vi "GetHWI.vi"(0 "NI Card in":refnum<class "NI Card.lvclass">, 11 "error in (no error)":errorcluster) -> (4 "NI Card out":refnum<class "NI Card.lvclass">, 6 "NI Card Hardware Image":T2, 8 "Parsed data":T1(array[cluster]), 15 "error out":errorcluster)   [LabVIEW 2013, in "NI Card.lvclass"]
uses:
  NI Card.lvclass
  NI Card.lvclass/NI Card.ctl
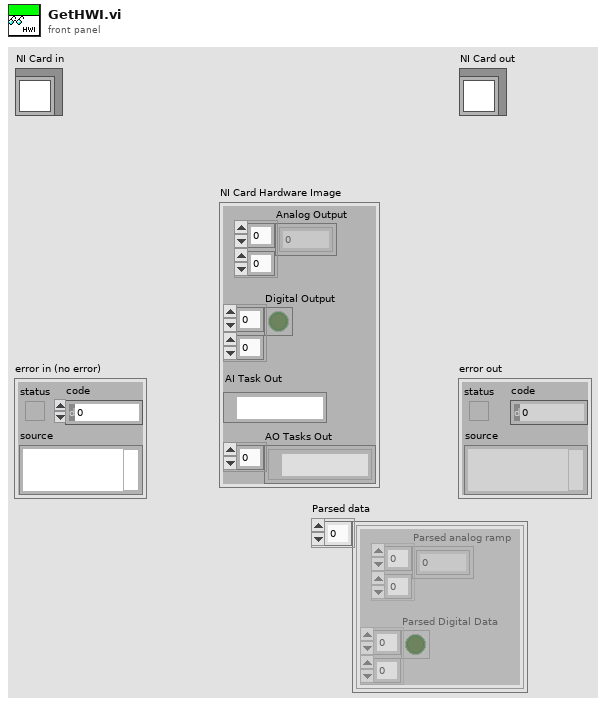
[diagram p1: front panel]
types:
  T1 = cluster{"Parsed analog ramp":dbl[][], "Parsed Digital Data":bool[][]}[]
  T2 = cluster{"Analog Output ":dbl[][], "Digital Output":bool[][], "AI Task Out":refnum<k21>, "AO Tasks Out":refnum<k21>[]}
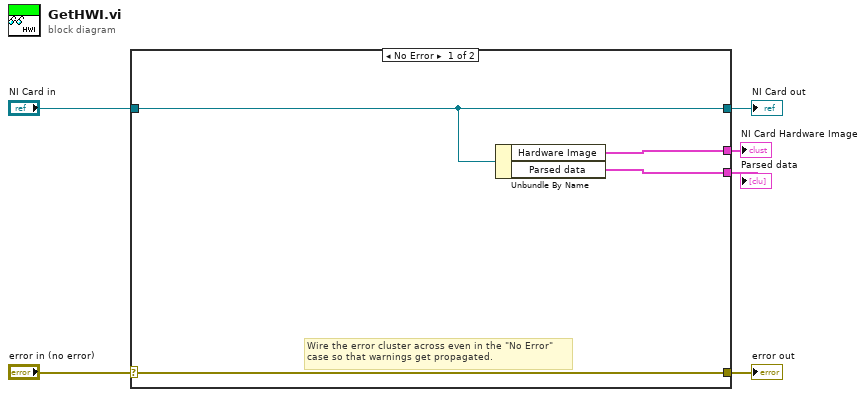
[diagram p0: block diagram]
diagram:
  n1 = case shown="No Error" "error in (no error)" {
    selector: "error in (no error)" -> [w10 w12]
    tunnel: [w10 w12] -> w5
    tunnel: [w9 w11] -> w3
    tunnel: "NI Card in" -> [w9 w11]
    tunnel: [w8 _] -> w2
    tunnel: [w7 _] -> w1
    frame No Error {
      # "Wire the error cluster across even in the \"No Error\"\ncase so that warnings get propagated."
      n2 = Unbundle By Name(w9) -> ("Hardware Image"=w8:T2, "Parsed data"=w7:T1)
    }
    frame Error {
    }
  }
  "error out" <- w5
  "NI Card out" <- w3
  "NI Card Hardware Image" <- w2
  "Parsed data" <- w1
